vi "Handle Error.vi"(8 "error in (no error)":errorcluster, 11 "CIFTemplatePlugin in":refnum<class "CIFTemplatePlugin.lvclass">) -> (0 "error out":errorcluster, 3 "CIFTemplatePlugin out":refnum<class "CIFTemplatePlugin.lvclass">)   [LabVIEW 2021, in "CIFTemplatePlugin.lvclass"]
uses:
  CIFTemplatePlugin.lvclass
  CIFTemplatePlugin.lvclass/CIFTemplatePlugin.ctl
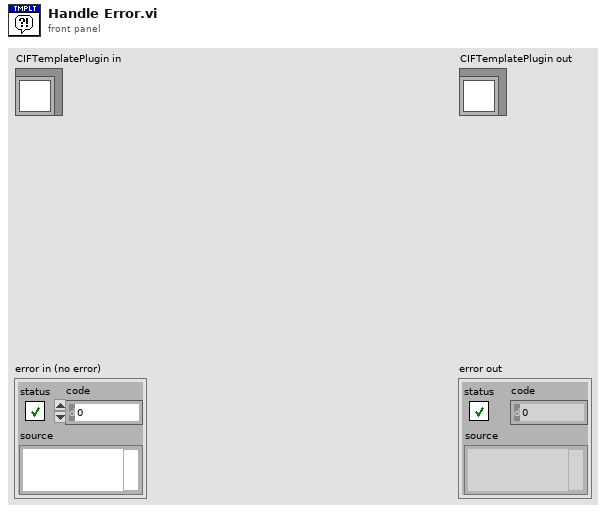
[diagram p1: front panel]
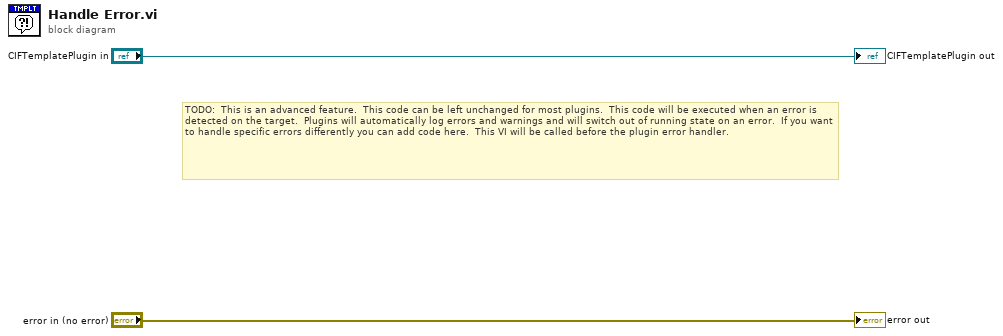
[diagram p0: block diagram]
diagram:
  # "TODO:  This is an advanced feature.  This code can be left unchanged for most plugins.  This code will be executed when an error is detected on the target.  Plugins will automatically log errors and warnings and will switch out of running state on an error.  If you want to handle specific errors differently you can add code here.  This VI will be called before the plugin error handler."
  "error out" <- "error in (no error)"
  "CIFTemplatePlugin out" <- "CIFTemplatePlugin in"
